vi "Split_DS_By_1cls.vi"() -> ()   [LabVIEW 2020]
uses:
  <vilib>/Utility/file.llb/Read Delimited Spreadsheet (string).vi
panel:
  out "new path":path
  out "error out 2":errorcluster
  out "error out":errorcluster
  out "Numeric":i32
  out "cancelled":bool
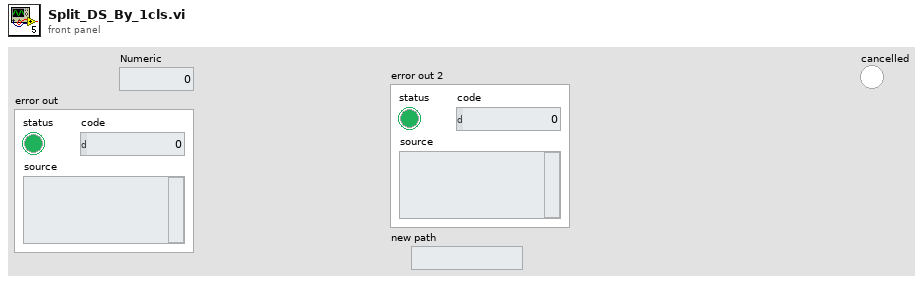
[diagram p1: front panel]
types:
  T1 = typedef "IMAQ Image.ctl" = refnum<image>
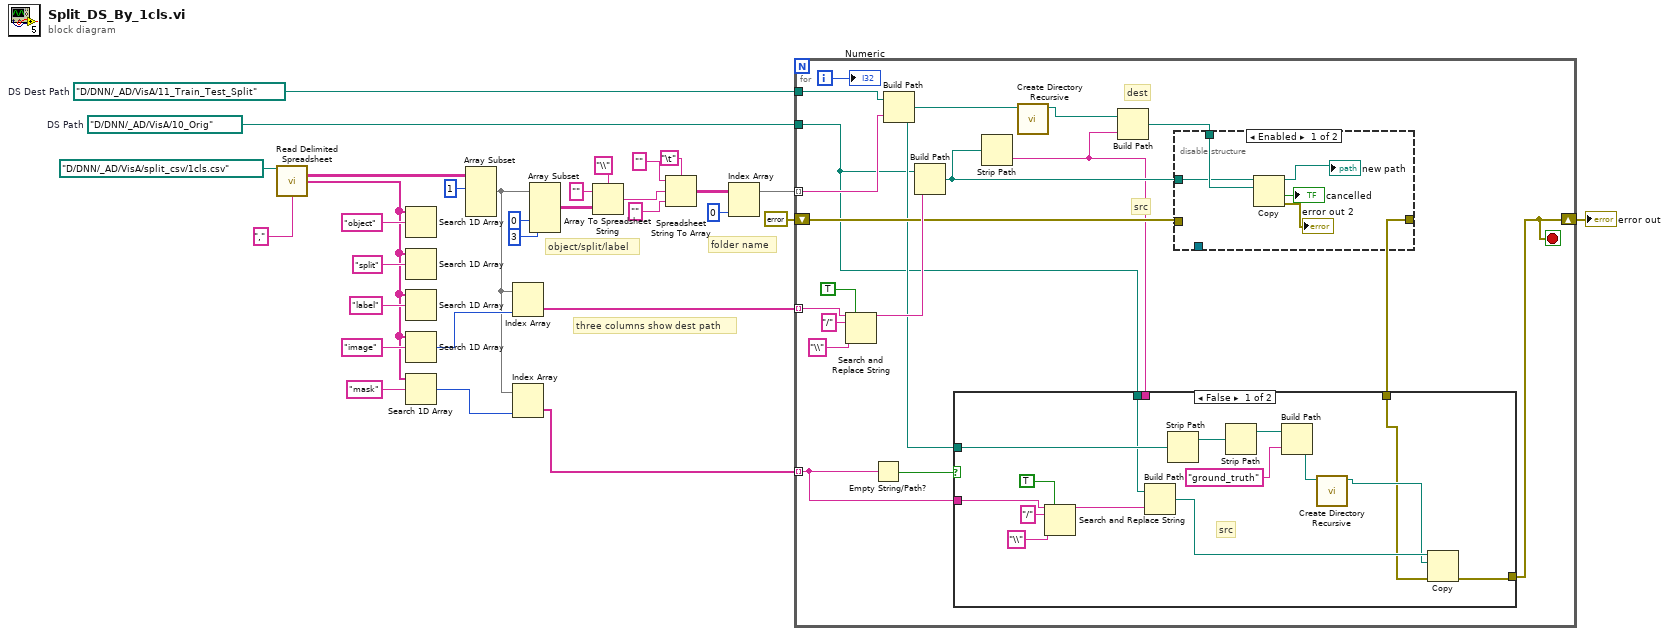
[diagram p0: block diagram]
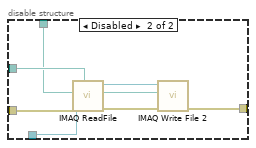
[diagram p3: hidden frame]
diagram:
  w12 = path "D:/DNN/_AD/VisA/11_Train_Test_Split"  # DS Dest Path
  w6 = path "D:/DNN/_AD/VisA/10_Orig"  # DS Path
  # "object/split/label"
  # "folder name"
  # "three columns show dest path"
  n1 = call-poly <vilib>:"Read Delimited Spreadsheet.vi"("file path (dialog if empty)"=path "D:/DNN/_AD/VisA/split_csv/1cls.csv", "delimiter (\\t)"="," ("delimiter (\\t)")) -> ("all rows"=w22:string[][], "first row"=w24:string[])  [unwired: 8 in, 4 out]
  n2 = Search 1D Array(1D array=w24, element="object") -> ()  [unwired: 1 in, 1 out]
  n3 = Search 1D Array(1D array=w24, element="split") -> ()  [unwired: 1 in, 1 out]
  n4 = Search 1D Array(1D array=w24, element="label") -> ()  [unwired: 1 in, 1 out]
  n5 = Search 1D Array(1D array=w24, element="image") -> (index of element=w8:i32)  [unwired: 1 in]
  n6 = Search 1D Array(1D array=w24, element="mask") -> (index of element=w2:i32)  [unwired: 1 in]
  n7 = Array Subset(array=w22, index (row)=1 ("index")) -> (w3:string[][])  [unwired: 3 in]
  n8 = Index Array(array=w3, index (col)=w8) -> (element=w7:string[])  [unwired: 1 in]
  n9 = Index Array(array=w3, index (col)=w2) -> (element=w1:string[])  [unwired: 1 in]
  n10 = Array Subset(array=w3, index (col)=0 ("index"), length (col)=3 ("length")) -> (w19:string[][])  [unwired: 2 in]
  n11 = Array To Spreadsheet String(delimiter (Tab)="\\", array=w19, 3:"" ("format string")) -> (spreadsheet string=w13:string)
  n12 = Spreadsheet String To Array(delimiter (Tab)="\t", format string="" ("spreadsheet string"), spreadsheet string=w13, array type (2D Dbl)="" ("spreadsheet string")) -> (array=w11:string[][])
  n13 = Index Array(array=w11, index (col)=0 ("disabled index (col)")) -> (element=w10:string[])  [unwired: 1 in]
  n14 = for {
    tunnel: w10 -> [w49] mode=indexing
    tunnel: w12 -> [w50]
    tunnel: w7 -> [w48] mode=indexing
    tunnel: w6 -> [w36]
    shift-right: [w32] -> w4
    shift-left: errorcluster {"status"=FALSE, "code"=0, "source"=""} ("error out") -> [w41]
    tunnel: w1 -> [w35] mode=indexing
    i -> [w43]
    stop <- w32 stop-if-true
    # "src"
    # "dest"
    n15 = Search and Replace String(replace all?=TRUE ("replace all? (F)"), input string=w48, search string="/", replace string="\\" ("replace string (\"\")")) -> (result string=w44:string)  [unwired: 4 in, 3 out]
    n16 = Empty String/Path?(string/path=w35) -> (empty?=w34:bool)
    n17 = Build Path(base path=w50, name or relative path=w49) -> (appended path=w37:path)
    n18 = Build Path(base path=w36, name or relative path=w44) -> (appended path=w42:path)
    n19 = Strip Path(path=w42) -> (name=w38:string)  [unwired: 1 out]
    n20 = call <vilib>:"Create Directory Recursive.vi"("directory"=w37) -> ("directory copy"=w40:path)  [unwired: 4 in, 2 out]
    n21 = Build Path(base path=w40, name or relative path=w38) -> (appended path=w39:path)
    n22 = disable-structure shown="Enabled" {
      disable-tunnel: w39 -> [w69 w72]
      disable-tunnel: w42 -> [w68 w77]
      disable-tunnel: _ -> [_ w78]
      disable-tunnel: [_ w74] -> w33
      disable-tunnel: w41 -> [_ w73]
      frame Enabled {
        n23 = Copy(10:w69, 11:w68) -> (0:→"error out 2":errorcluster, 1:→"cancelled":bool, 3:→"new path":path)  [unwired: 3 in]
      }
      frame Disabled {
        n24 = call "IMAQ ReadFile"("File Path"=w77, "error in (no error)"=w73, "Image"=w78) -> ("error out"=w75:errorcluster, "Image Out"=w76:T1)  [unwired: 4 in, 3 out]
        n25 = call-poly "IMAQ Write File 2"("error in (no error)"=w75, "File Path"=w72, "Image"=w76) -> ("error out"=w74:errorcluster)  [unwired: 7 in, 1 out]
      }
    }
    n26 = case shown="False" w34 {
      tunnel: w38 -> [_ _]
      tunnel: w37 -> [w65 _]
      tunnel: w36 -> [w61 _]
      tunnel: w35 -> [w56 _]
      tunnel: w33 -> [w51 w66]
      tunnel: [w52 w66] -> w32
      frame False {
        # "src"
        n27 = Search and Replace String(replace all?=TRUE ("replace all? (F)"), input string=w56, search string="/", replace string="\\" ("replace string (\"\")")) -> (result string=w55:string)  [unwired: 4 in, 3 out]
        n28 = Build Path(base path=w61, name or relative path=w55) -> (appended path=w54:path)
        n29 = Strip Path(path=w65) -> (stripped path=w64:path)  [unwired: 1 out]
        n30 = Strip Path(path=w64) -> (stripped path=w63:path)  [unwired: 1 out]
        n31 = Build Path(base path=w63, name or relative path="ground_truth" ("Image Name")) -> (appended path=w60:path)
        n32 = call <vilib>:"Create Directory Recursive.vi"("directory"=w60) -> ("directory copy"=w53:path)  [unwired: 4 in, 2 out]
        n33 = Copy(8:w51, 10:w53, 11:w54) -> (0:w52:errorcluster)  [unwired: 2 in, 2 out]
      }
      frame True {
      }
    }
    "Numeric" <- w43
  }
  "error out" <- w4
